vi "To Serial Form.vi"(6 "Serial Version":T1, 10 "Serializer in":refnum<class "Serializer.lvclass">, 11 "Instrument in":refnum<class "Instrument.lvclass">) -> (0 "error out":errorcluster, 2 "Serializer out":refnum<class "Serializer.lvclass">, 3 "Instrument out":refnum<class "Instrument.lvclass">)   [LabVIEW 2012]
uses:
  <userlib>/Serialization/Serializable/Serializable.lvclass
  <userlib>/Serialization/Serializable/Insert Boolean.vi
  <userlib>/Serialization/Serializer/Serializer.lvclass
  <userlib>/Serialization/Serialization Common/Serial Version.ctl
  <userlib>/Serialization/Serialization Common/Serialization Common.lvlib
  Instrument.lvclass
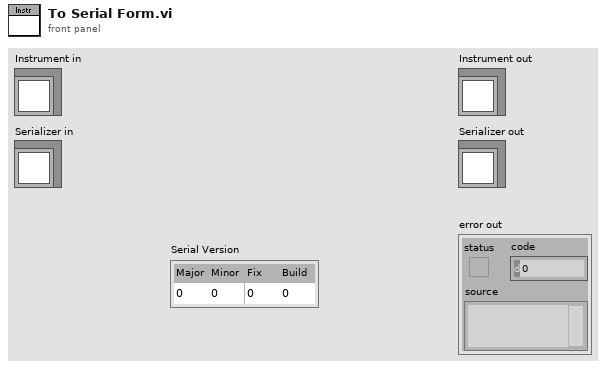
[diagram p1: front panel]
types:
  T1 = typedef "Serialization Common.lvlib/Serial Version.ctl" = cluster{"Major":u16, "Minor":u16, "Fix":u16, "Build":u16}
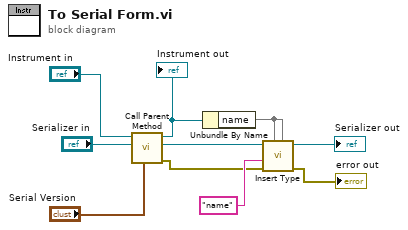
[diagram p0: block diagram]
diagram:
  n1 = call-parent "Call Parent Method"("Serial Version"="Serial Version", "Serializer in"="Serializer in", "Serializable in"="Instrument in") -> ("error out"=w4:errorcluster, "Serializer out"=w3:refnum<class "Serializer.lvclass">, "Serializable out"=w7:refnum<class "Serializable.lvclass">)  [unwired: 6 in]
  "Instrument out" <- w7
  n2 = Unbundle By Name(w7) -> ("name"=w6)
  n3 = call-poly <userlib>:"Insert Type.vi"("Boolean"=w6, "Default Value"=w6, "error in (no error)"=w4, "Name"="name", "Serializer in"=w3) -> ("error out"=→"error out":errorcluster, "Serializer out"=→"Serializer out":refnum<class "Serializer.lvclass">)  [unwired: 5 in]
